vi "JSONtext-test-results-20210421.vi"() -> ()   [LabVIEW 2019]
panel:
  out "XY Graph":cluster{dbl[], dbl[]}[](graph)=[{[8e-06, 2.5298221281347037e-05, 8e-05, 0.00025298221281347036, 0.0008, 0.0025298221281347035, 0.008, 0.025298221281347035, 0.08, 0.25298221281347033, 0.8, 2.529822128134703, 8.0, 25.298221281347036, 80.0], [0.00024199999461416155, 0.00012849999620812014, 0.00013020000187680125, 0.00012209999840706587, 0.00012589999823831022, 0.00012109999806853011, 0.0001238999975612387, 0.00012900000001536682, 0.00017829999706009403, 0.00021320000087143853, 0.0002686000007088296, 0.0003947000004700385, 0.000727099999494385, 0.0014905999996699393, 0.004119099998206366]}, {[8e-06, 2.5298221281347037e-05, 8e-05, 0.00025298221281347036, 0.0008, 0.0025298221281347035, 0.008, 0.025298221281347035, 0.08, 0.25298221281347033, 0.8, 2.529822128134703, 8.0, 25.298221281347036, 80.0], [7.550000009359792e-05, 9.370000043418258e-05, 5.589999636868015e-05, 5.389999569160864e-05, 5.450000026030466e-05, 5.2299998060334474e-05, 5.400000372901559e-05, 5.4899996030144393e-05, 7.139999797800556e-05, 9.919999865815043e-05, 0.00014229999942472205, 0.00014830000145593658, 0.00015339999663410708, 0.00018339999951422215, 0.00021359999664127827]}, {[8e-06, 2.5298221281347037e-05, 8e-05, 0.00025298221281347036, 0.0008, 0.0025298221281347035, 0.008, 0.025298221281347035, 0.08, 0.25298221281347033, 0.8, 2.529822128134703, 8.0, 25.298221281347036, 80.0], [0.00013020000187680125, 0.00010710000060498714, 0.00011150000500492752, 0.0001345000055152923, 0.00021379999816417694, 0.00045060000411467627, 0.0011432999963290058, 0.0129947000023094, 0.014772700000321493, 0.050064700000802986, 0.1260007000018959, 0.3630429999975604, 1.2440353000056348, 3.6396440000025905, 11.487841600006504]}, {[8e-06, 2.5298221281347037e-05, 8e-05, 0.00025298221281347036, 0.0008, 0.0025298221281347035, 0.008, 0.025298221281347035, 0.08, 0.25298221281347033, 0.8, 2.529822128134703, 8.0, 25.298221281347036, 80.0], [8.689999958733097e-05, 6.830000347690657e-05, 7.079999340930954e-05, 0.00011819999781437218, 0.00016630000027362257, 0.00036859999818261713, 0.001043800002662465, 0.0032257999991998076, 0.014601800001400989, 0.0554649999976391, 0.1594076999972458, 0.36541720000241185, 1.0837763999952585, 3.921743899998546, 16.2716803000003]}, {[8e-06, 2.5298221281347037e-05, 8e-05, 0.00025298221281347036, 0.0008, 0.0025298221281347035, 0.008, 0.025298221281347035, 0.08, 0.25298221281347033, 0.8, 2.529822128134703, 8.0, 25.298221281347036, 80.0], [0.0005345999961718917, 0.00039760000072419643, 0.00036839999665971845, 0.000428699997428339, 0.0005604999969364144, 0.000992599998426158, 0.002365000000281725, 0.01640439999755472, 0.02962419999676058, 0.10584209999797167, 0.28581929999927524, 0.7290032000018982, 2.328692199997022, 7.563061900000321, 27.76385460000165]}]
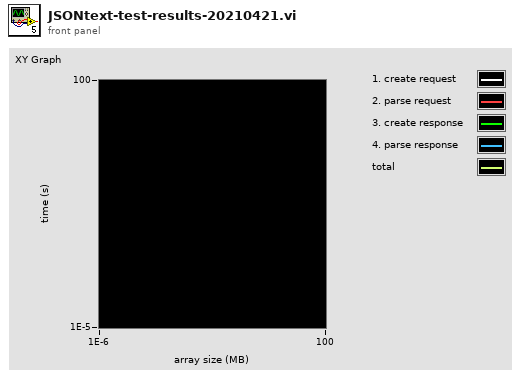
[diagram p1: front panel]
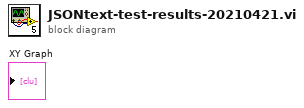
[diagram p0: block diagram]
diagram:
